vi "AsyncCall.vi"(9 "ErrorQueue":refnum<queue>, 10 "PreSetupQueue":refnum<queue>, 11 "Actor":refnum<class "Actor.lvclass">) -> ()   [LabVIEW 2020, in "jettl.lvlib"]
uses:
  jettl.lvlib
  Base/ConcreteActor/ConcreteActor.lvclass
  Actor/Actor.lvclass
  Lifecycle.ctl
  PreSetup.ctl
  TellOrigin.ctl
  MessageMetadata.ctl
panel:
  in  "Error in 2":errorcluster
  out "Error out 2":errorcluster
  in  "Teller 2":T1 {"AbsoluteTime" format="%<%x %.3X>T"}
  out "ConcreteActor 4":refnum<class "ConcreteActor.lvclass">
  in  "ConcreteActor 3":refnum<class "ConcreteActor.lvclass">
  in  "Error in":errorcluster
  out "Error out":errorcluster
  in  "Error":errorcluster
  in  "Teller":T1 {"AbsoluteTime" format="%<%x %.3X>T"}
  in  "Actor 2":refnum<class "Actor.lvclass">
  out "ConcreteActor":refnum<class "ConcreteActor.lvclass">
  in  "ConcreteActor 2":refnum<class "ConcreteActor.lvclass">
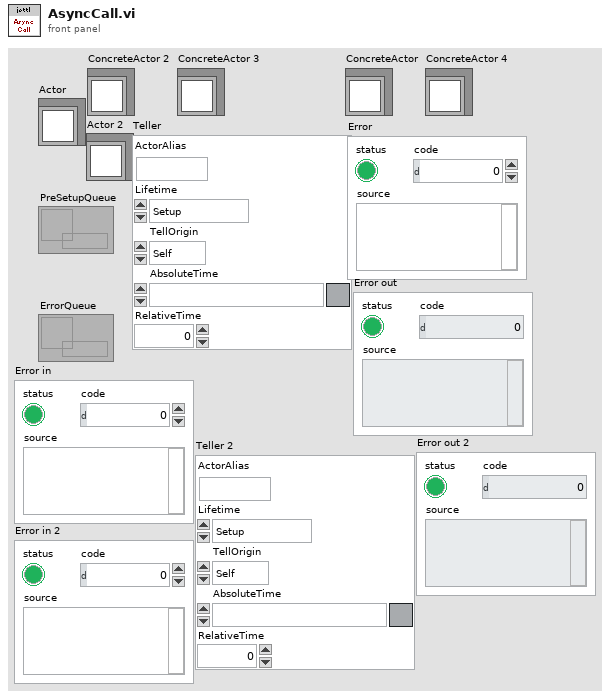
[diagram p1: front panel]
types:
  T1 = typedef "jettl.lvlib/MessageMetadata.ctl" = cluster{"ActorAlias":string, "Lifetime":T2, "TellOrigin":T3, "AbsoluteTime":timestamp, "RelativeTime":dbl}
  T2 = typedef "jettl.lvlib/Lifecycle.ctl" = enum16{"Setup", "TeardownBeforeStart", "Start", "Running", "Stop", "TeardownAfterStart"}
  T3 = typedef "jettl.lvlib/TellOrigin.ctl" = enum16{"Self", "Mediator", "Component"}
  T4 = typedef "jettl.lvlib/Lifetime.ctl" = enum16{"Init", "Spawn", "Setup", "TeardownBeforeRunning", "Running", "StopCalled", "StoppingWithComponents", "StoppingNoComponents", "TeardownAfterRunning", "Stopped"}
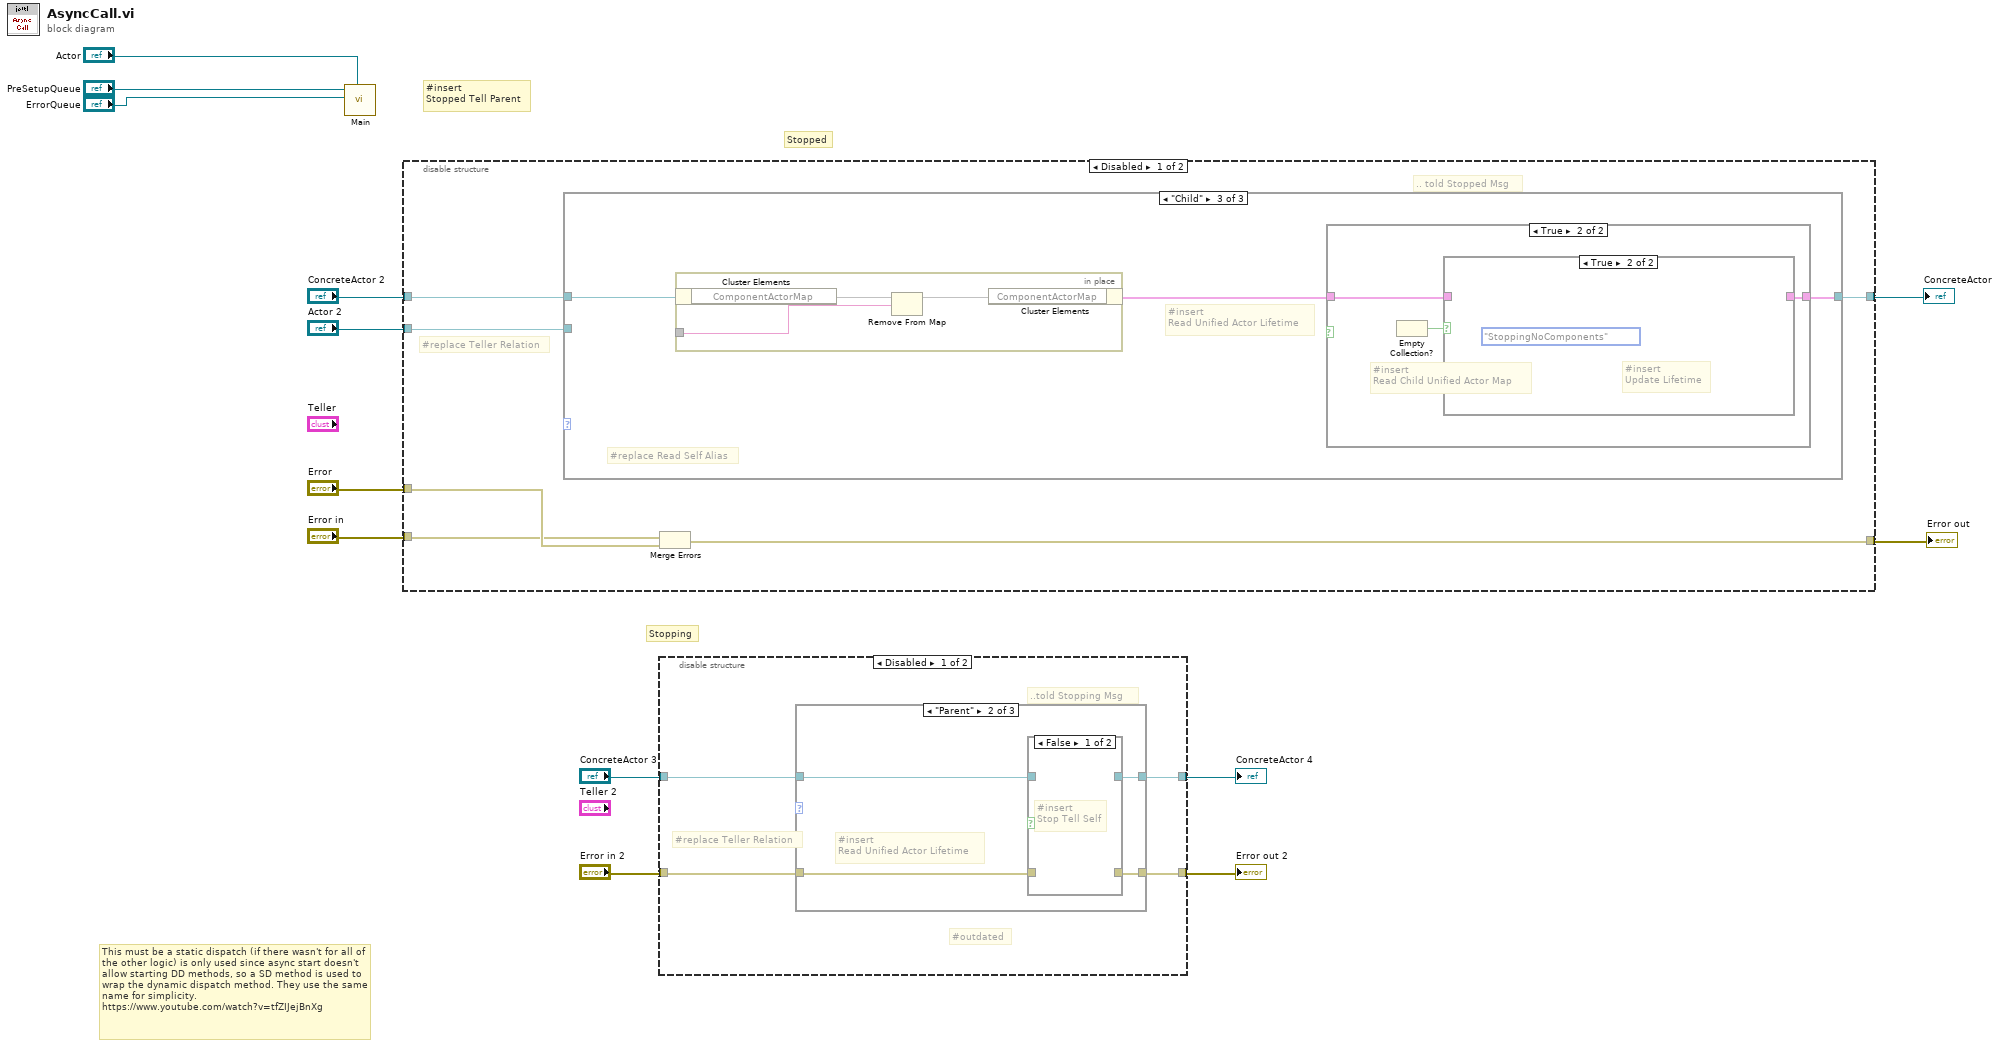
[diagram p0: block diagram]
diagram:
  # "Stopped"
  # "Stopping"
  # "#insert\nStopped Tell Parent"
  # "This must be a static dispatch (if there wasn't for all of the other logic) is only used since async start doesn't allow starting DD methods, so a SD method is used to wrap the dynamic dispatch method. They use the same name for simplicity.\nhttps://www.youtube.com/watch?v=tfZIJejBnXg"
  n1 = call-dynamic "Main.vi"("Actor"="Actor", "ErrorQueue"="ErrorQueue", "PreSetupQueue"="PreSetupQueue") -> ()  [unwired: 7 in, 2 out]
  n2 = disable-structure shown="Disabled" {
    disable-tunnel: [w19 w37] -> w10
    disable-tunnel: "ConcreteActor 2" -> [w18 w37]
    disable-tunnel: "Actor 2" -> [w17 _]
    disable-tunnel: "Error" -> [w16 _]
    disable-tunnel: "Error in" -> [w15 w38]
    disable-tunnel: [w14 w38] -> w5
    frame Disabled {
      # "#replace Teller Relation"
      # ".. told Stopped Msg"
      n3 = case shown="\"Child\"" {
        selector: _ -> [_ _ _]
        tunnel: w18 -> [w20 w21 w23]
        tunnel: [w20 w21 w25] -> w19
        tunnel: w17 -> [_ _ w24]
        frame "Self" {
          # "Case will not fundamentally execute"
        }
        frame "Parent" {
          # "Case will not fundamentally execute"
        }
        frame "Child" {
          # "#insert\nRead Unified Actor Lifetime"
          # "#replace Read Self Alias"
          n4 = in-place {
            in-place-border: [w28] -> _
            n5 = in-place-cluster #1(w23) -> ("ComponentActorMap"=w27)
            n6 = Remove From Map(11:w27) -> (3:w26:map{string, i32}, 10:w28:string)  [unwired: 2 out]
            n7 = in-place-cluster #1("ComponentActorMap"=w26) -> (w22:cluster{})
          }
          n8 = case shown="True" {
            selector: _ -> [_ _]
            tunnel: w22 -> [w29 w30]
            tunnel: [w29 w32] -> w25
            frame False {
            }
            frame True {
              # "#insert\nRead Child Unified Actor Map"
              n9 = Empty Collection?() -> (0:w31:bool)  [unwired: 1 in]
              n10 = case shown="True" w31 {
                tunnel: [w33 w34] -> w32
                tunnel: w30 -> [w33 w35]
                frame False {
                }
                frame True {
                  w36 = Lifetime."StoppingNoComponents" ("Lifetime")
                  # "#insert\nUpdate Lifetime"
                }
              }
            }
          }
        }
      }
      n11 = Merge Errors(w15, w16) -> (w14:errorcluster)
    }
    frame Enabled {
    }
  }
  "ConcreteActor" <- w10
  "Error out" <- w5
  n12 = disable-structure shown="Disabled" {
    disable-tunnel: "ConcreteActor 3" -> [w42 w57]
    disable-tunnel: [w41 w57] -> w3
    disable-tunnel: "Error in 2" -> [w40 w56]
    disable-tunnel: [w39 w56] -> w1
    frame Disabled {
      # "#outdated"
      # "#replace Teller Relation"
      # "..told Stopping Msg"
      n13 = case shown="\"Parent\"" {
        selector: _ -> [_ _ _]
        tunnel: w42 -> [w44 w45 w55]
        tunnel: [w44 w48 w55] -> w41
        tunnel: w40 -> [w43 w47 w54]
        tunnel: [w43 w46 w54] -> w39
        frame "Self" {
          # "Case will not fundamentally execute"
        }
        frame "Parent" {
          # "#insert\nRead Unified Actor Lifetime"
          n14 = case shown="False" {
            selector: _ -> [_ _]
            tunnel: [w51 w53] -> w48
            tunnel: w47 -> [w50 w52]
            tunnel: [_ w52] -> w46
            tunnel: w45 -> [w49 w53]
            frame False {
              # "#insert\nStop Tell Self"
            }
            frame True {
            }
          }
        }
        frame "Child" {
          # "Case will not fundamentally execute"
        }
      }
    }
    frame Enabled {
    }
  }
  "ConcreteActor 4" <- w3
  "Error out 2" <- w1
